vi "MeasureStub.vi"(6 "Graph in":cluster{dbl[], dbl[]}, 7 "XY Graph":refnum<vi>, 8 "error in":errorcluster, 10 "Reference Cell":i32) -> (0 "error out":errorcluster, 1 "Values":cluster{dbl[], dbl[]}, 2 "P1/P2":dbl format="%#_13g")   [LabVIEW 2013]
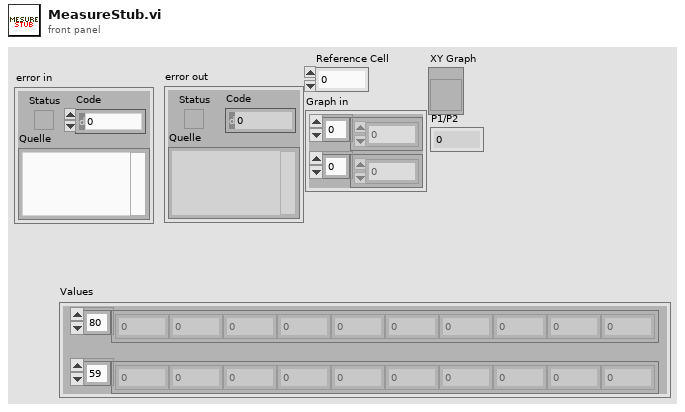
[diagram p1: front panel]
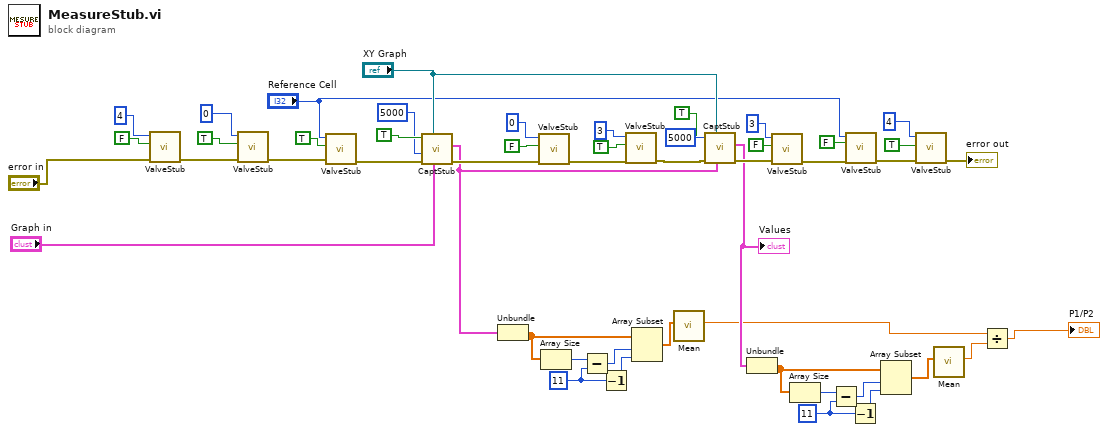
[diagram p0: block diagram]
diagram:
  w8 = 11
  w13 = 11
  n1 = call "ValveStub.vi"("error in"="error in", "ON"=FALSE, "Valve"=4) -> ("error out"=w46:errorcluster)  [unwired: 8 in]
  n2 = call "ValveStub.vi"("error in"=w46, "ON"=TRUE, "Valve"=0) -> ("error out"=w45:errorcluster)  [unwired: 8 in]
  n3 = call "ValveStub.vi"("error in"=w45, "ON"=TRUE, "Valve"="Reference Cell") -> ("error out"=w39:errorcluster)  [unwired: 8 in]
  n4 = call "CaptStub.vi"("Graph in"="Graph in", "XY Graph"="XY Graph", "error in"=w39, "Length"=5000, "ON"=TRUE) -> ("error out"=w34:errorcluster, "Values"=w6:cluster{dbl[], dbl[]})  [unwired: 5 in]
  n5 = Unbundle(w6) -> (w17:dbl[])  [unwired: 1 out]
  n6 = call "ValveStub.vi"("error in"=w34, "ON"=FALSE, "Valve"=0) -> ("error out"=w35:errorcluster)  [unwired: 8 in]
  n7 = Array Size(array=w17) -> (size(s)=w16:i32)
  n8 = Subtract(x=w16, y=w13) -> (x-y=w15:i32)
  n9 = Decrement(x=w13) -> (x-1=w14:i32)
  n10 = call "ValveStub.vi"("error in"=w35, "ON"=TRUE, "Valve"=3) -> ("error out"=w28:errorcluster)  [unwired: 8 in]
  n11 = Array Subset(array=w17, index=w15, length=w14) -> (w1:dbl[])
  n12 = call "Mean.vi"("Array"=w1) -> ("Mean"=w2:dbl)  [unwired: 10 in]
  n13 = call "CaptStub.vi"("Graph in"=w6, "XY Graph"="XY Graph", "error in"=w28, "Length"=5000, "ON"=TRUE) -> ("error out"=w27:errorcluster, "Values"=w7:cluster{dbl[], dbl[]})  [unwired: 5 in]
  "Values" <- w7
  n14 = Unbundle(w7) -> (w12:dbl[])  [unwired: 1 out]
  n15 = call "ValveStub.vi"("error in"=w27, "ON"=FALSE, "Valve"=3) -> ("error out"=w24:errorcluster)  [unwired: 8 in]
  n16 = Array Size(array=w12) -> (size(s)=w11:i32)
  n17 = Subtract(x=w11, y=w8) -> (x-y=w10:i32)
  n18 = call "ValveStub.vi"("error in"=w24, "ON"=FALSE, "Valve"="Reference Cell") -> ("error out"=w21:errorcluster)  [unwired: 8 in]
  n19 = Decrement(x=w8) -> (x-1=w9:i32)
  n20 = Array Subset(array=w12, index=w10, length=w9) -> (w4:dbl[])
  n21 = call "ValveStub.vi"("error in"=w21, "ON"=TRUE, "Valve"=4) -> ("error out"=→"error out":errorcluster)  [unwired: 8 in]
  n22 = call "Mean.vi"("Array"=w4) -> ("Mean"=w3:dbl)  [unwired: 10 in]
  n23 = Divide(x=w2, y=w3) -> (x/y=→"P1/P2":dbl)
